vi "SubVI_PupilDetection_image_and_parameters_in_info_and_image_out.vi"(0 "Image":picture, 4 "img_cols":u16, 5 "img_rows":u16, 6 "u8Image":u8[](array[numeric])) -> (12 "output image":picture, 13 "Image to save":u8[][](array[numeric]))   [LabVIEW 2021]
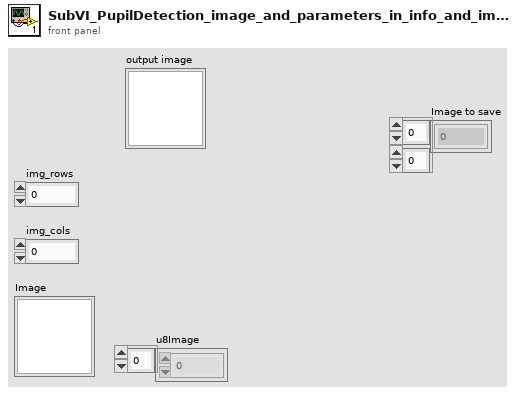
[diagram p1: front panel]
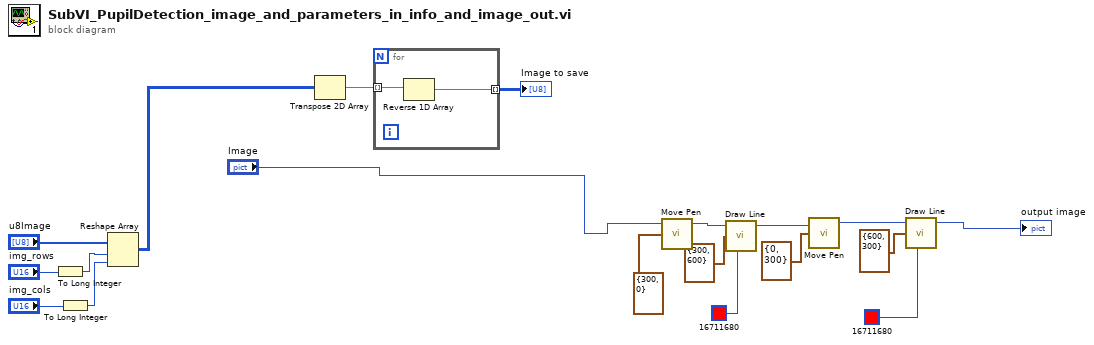
[diagram p0: block diagram]
diagram:
  n1 = To Long Integer(number="img_rows") -> (32bit integer=w13:i32)
  n2 = To Long Integer(number="img_cols") -> (32bit integer=w12:i32)
  n3 = Reshape Array("u8Image", w13, w12) -> (w11:u8[][])
  n4 = Transpose 2D Array(2D array=w11) -> (transposed array=w15:u8[][])
  n5 = for {
    tunnel: w15 -> [w21] mode=indexing
    tunnel: [w20] -> w14 mode=indexing
    n6 = Reverse 1D Array(array=w21) -> (reversed array=w20:u8[])
  }
  "Image to save" <- w14
  n7 = call <vilib>:"Move Pen.vi"("new position"=cluster{"x":i16, "y":i16} {"x"=300, "y"=0}, "picture"="Image") -> ("new picture"=w6:picture)  [unwired: 3 in]
  n8 = call <vilib>:"Draw Line.vi"("picture"=w6, "end point"=cluster{"x":i16, "y":i16} {"x"=300, "y"=600}, "color(black)"=u32 16711680) -> ("new picture"=w4:picture)  [unwired: 6 in]
  n9 = call <vilib>:"Move Pen.vi"("new position"=cluster{"x":i16, "y":i16} {"x"=0, "y"=300}, "picture"=w4) -> ("new picture"=w3:picture)  [unwired: 3 in]
  n10 = call <vilib>:"Draw Line.vi"("picture"=w3, "end point"=cluster{"x":i16, "y":i16} {"x"=600, "y"=300}, "color(black)"=u32 16711680) -> ("new picture"=→"output image":picture)  [unwired: 6 in]
